vi "SwissSPAD Live_Gate Configuration Storage.vi"(7 "Preset Configuration Refnum":refnum<vi>, 8 "Error In":errorcluster, 9 "Action":T1, 10 "Gate Configuration Definition in":T2, 11 "Gate Configuration Name in":string) -> (0 "Error Out":errorcluster, 1 "Configuration ID":i32, 2 "Gate Configuration Definition out":T2, 3 "Gate Configuration Name out":string, 4 "Gate Configuration Found?":bool, 5 "Gate Definition Found?":bool)   [LabVIEW 2021]
uses:
  SwissSPAD Live_SS2 Gate Configuration.ctl
  SwissSPAD Live_SS2 Gate Definition.ctl
  SwissSPAD Live_Gate Configuration Action.ctl
  SwissSPAD Live_Globals.vi
  <vilib>/UserTags/UserTags.lvlib
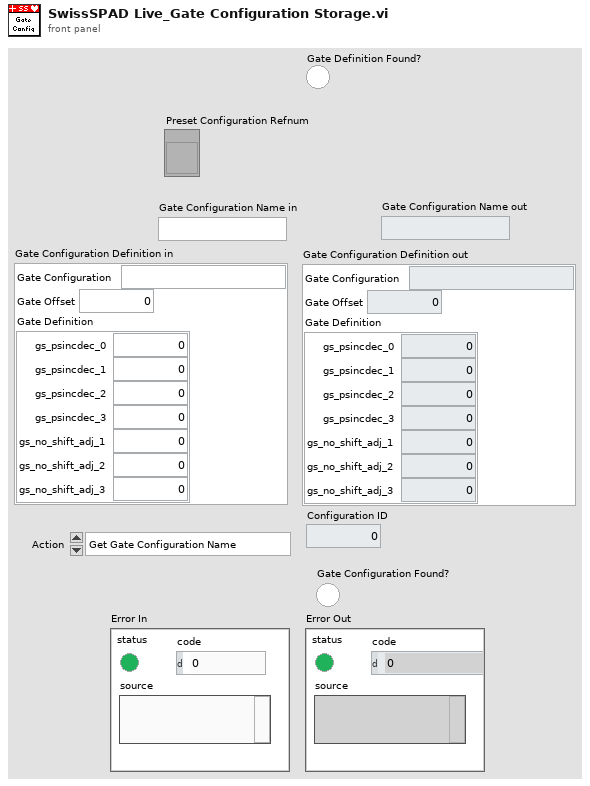
[diagram p1: front panel]
types:
  T1 = typedef "SwissSPAD Live_Gate Configuration Action.ctl" = enum16{"Get Gate Configuration Name", "Get Configuration by Name", "Add Gate Configuration", "Delete Gate Configuration", "Rename Gate Configuration"}
  T2 = typedef "SwissSPAD Live_SS2 Gate Configuration.ctl" = cluster{"Gate Configuration":string, "Gate Offset":u32, "Gate Definition":T3}
  T3 = typedef "SwissSPAD Live_SS2 Gate Definition.ctl" = cluster{"gs_psincdec_0":u32, "gs_psincdec_1":u32, "gs_psincdec_2":u32, "gs_psincdec_3":u32, "gs_no_shift_adj_1":u32, "gs_no_shift_adj_2":u32, "gs_no_shift_adj_3":u32}
  T4 = enum16{"Left Button", "Center Button", "Right Button", "Window Close"}
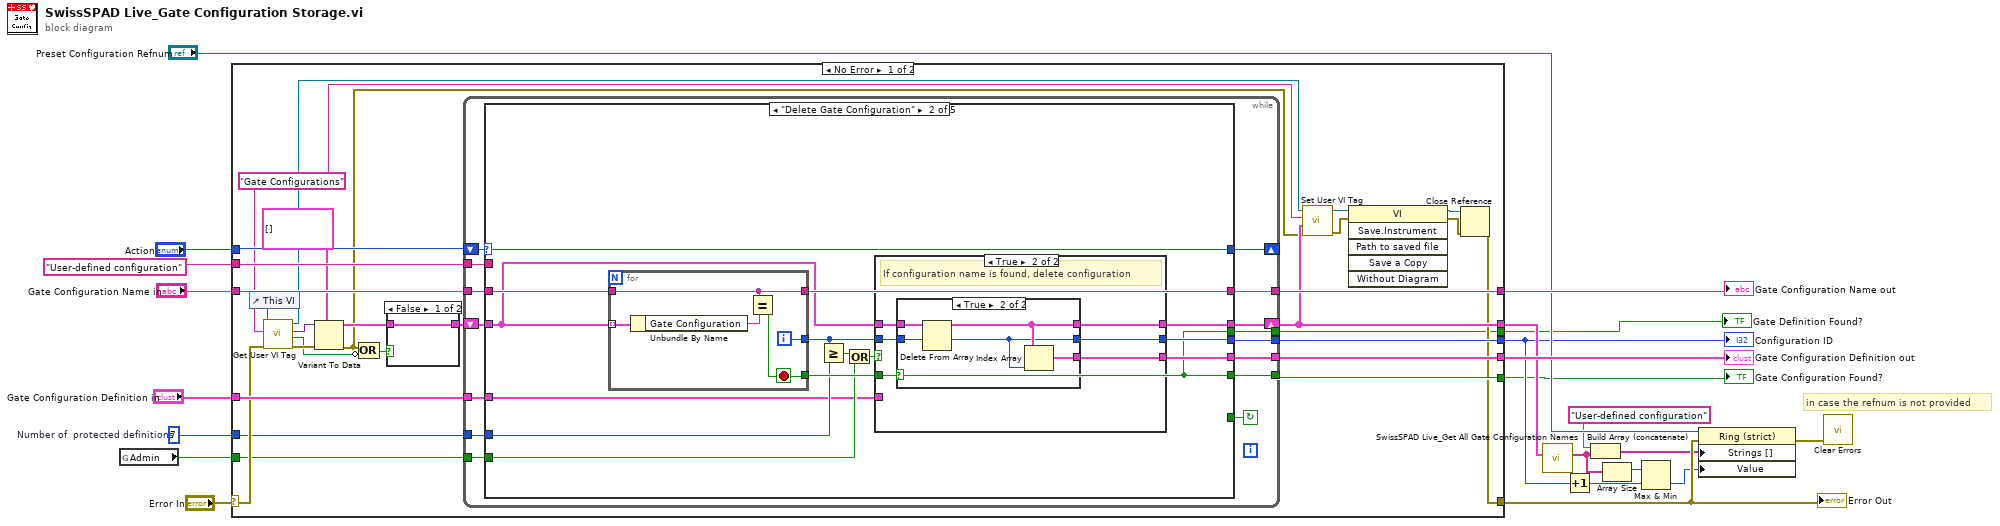
[diagram p0: block diagram]
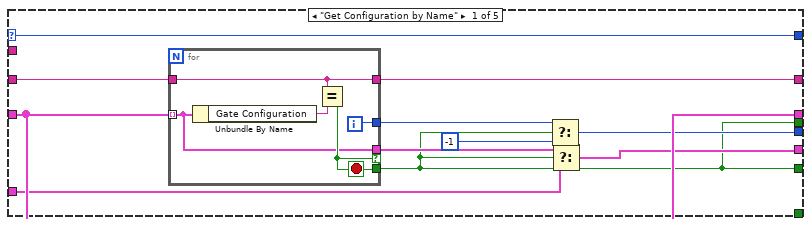
[diagram p3: hidden frame]
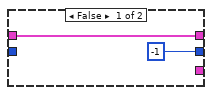
[diagram p5: hidden frame]
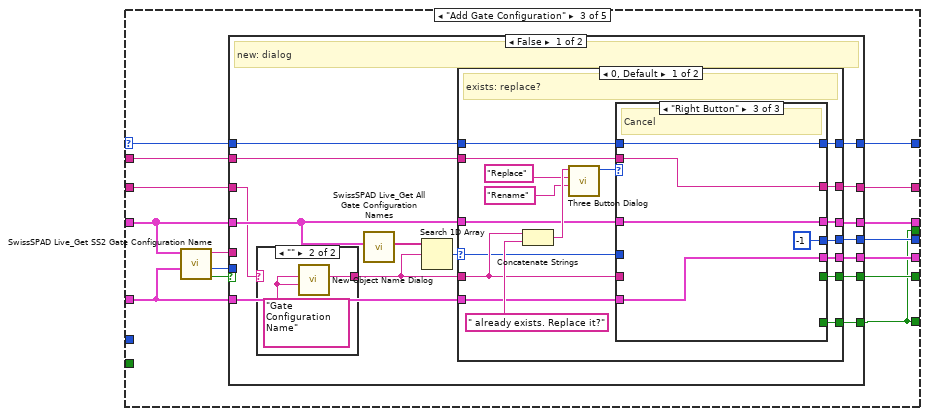
[diagram p6: hidden frame]
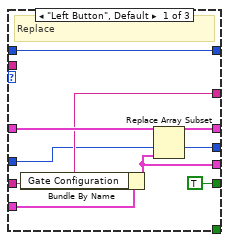
[diagram p8: hidden frame]
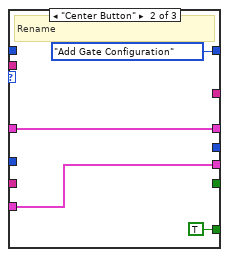
[diagram p9: hidden frame]
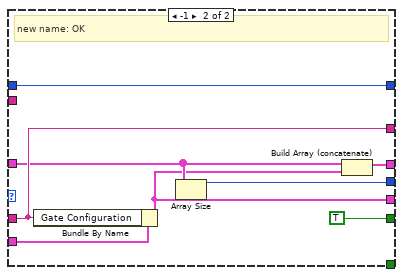
[diagram p10: hidden frame]
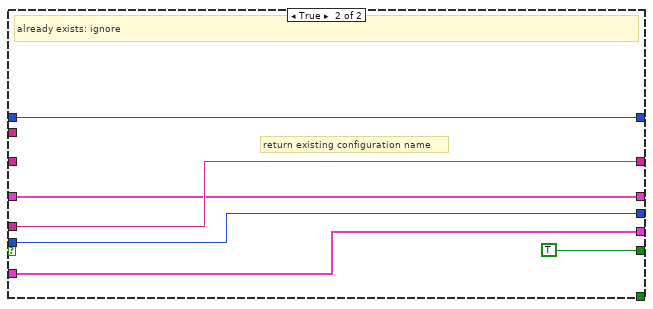
[diagram p11: hidden frame]
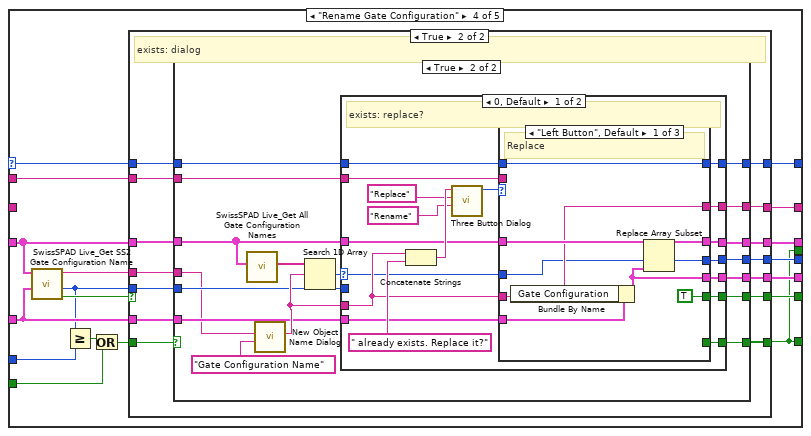
[diagram p12: hidden frame]
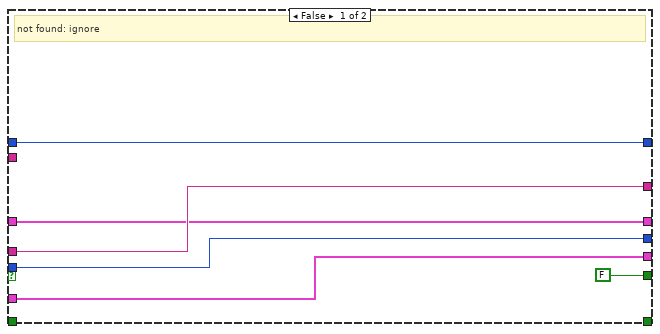
[diagram p13: hidden frame]
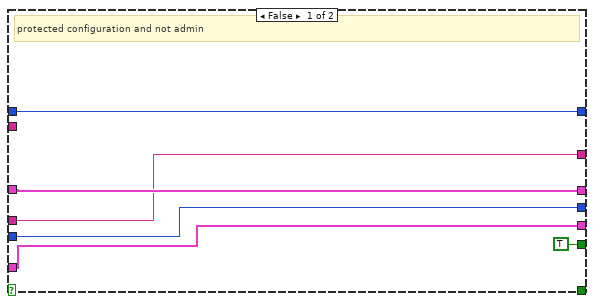
[diagram p14: hidden frame]
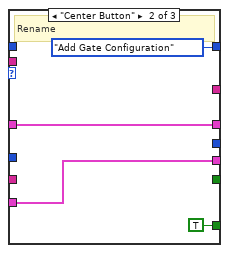
[diagram p15: hidden frame]
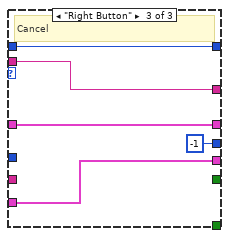
[diagram p16: hidden frame]
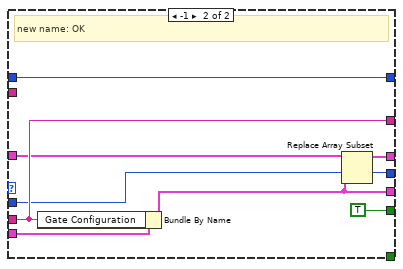
[diagram p17: hidden frame]
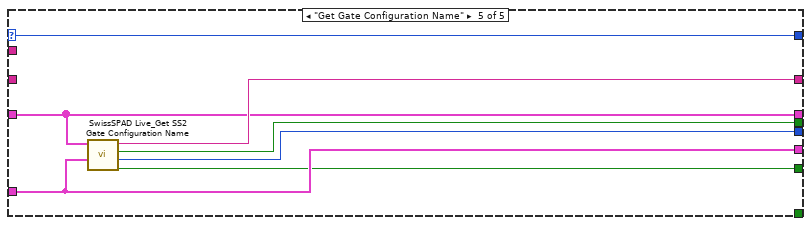
[diagram p18: hidden frame]
diagram:
  w6 = 7  # Number of  protected definitions
  # "in case the refnum is not provided"
  n1 = global read "SwissSPAD Live_Globals.vi" "Admin"() -> (w5:bool)
  n2 = case shown="No Error" "Error In" {
    selector: "Error In" -> [w28 w311]
    tunnel: "Action" -> [w51 _]
    tunnel: "Gate Configuration Name in" -> [w50 _]
    tunnel: [w49 _] -> w20
    tunnel: [w48 _] -> w19
    tunnel: "Gate Configuration Definition in" -> [w47 _]
    tunnel: [w46 _] -> w13
    tunnel: [w45 _] -> w14
    tunnel: "User-defined configuration" ("Object Name out") -> [w44 _]
    tunnel: [w37 _] -> w15
    tunnel: [w26 w311] -> w8
    tunnel: [w25 _] -> w9
    tunnel: w6 -> [w24 _]
    tunnel: w5 -> [w23 _]
    frame No Error {
      w35 = "Gate Configurations" ("Tag Name")
      n3 = control-ref of="This VI"() -> (w43:refnum<vi>)
      n4 = call <vilib>:"Get User VI Tag.vi"("error in (no error)"=w28, "Tag Name"=w35, "VI Refnum"=w43) -> ("error out"=w42:errorcluster, "Was Tag Found?"=w33:bool, "Value"=w41:variant, "dup VI Refnum"=w36:refnum<vi>)  [unwired: 5 in]
      n5 = Variant To Data(error in=w42, type=T2[] [] ("Array"), Variant=w41) -> (data=w39:T2[], error out=w27:errorcluster)
      n6 = Compound Arithmetic op=OR(w27, invert w33) -> (w34:bool)
      n7 = case shown="False" w34 {
        tunnel: w39 -> [w52 _]
        tunnel: [w52 _] -> w38
        frame False {
        }
        frame True {
        }
      }
      n8 = while {
        tunnel: w50 -> [w66]
        shift-right: [w61] -> w37
        shift-left: w38 -> [w65]
        tunnel: [w64] -> w46
        tunnel: [w63] -> w49
        tunnel: [w62] -> w48
        tunnel: w47 -> [w60]
        tunnel: [w59] -> w45
        shift-right: [w58] -> _
        shift-left: w51 -> [w67]
        tunnel: w44 -> [w56]
        tunnel: [w55] -> w25
        tunnel: w24 -> [w54]
        tunnel: w23 -> [w53]
        stop <- w57 continue-if-true
        n9 = case shown="\"Delete Gate Configuration\"" w67 {
          selector: w67 -> [w72 w93 w122 w208 w305]
          tunnel: w66 -> [w78 w97 w119 _ _]
          tunnel: w65 -> [w76 w95 w129 w214 w309]
          tunnel: [w68 w90 w123 w209 w307] -> w64
          tunnel: [w69 w91 w126 w211 w308] -> w63
          tunnel: [w77 w96 w130 w215 w310] -> w62
          tunnel: [w76 w94 w128 w213 w309] -> w61
          tunnel: w60 -> [w70 w84 w127 w212 w308]
          tunnel: [w74 w92 w124 w210 w306] -> w59
          tunnel: [w72 w93 w121 w207 w305] -> w58
          tunnel: [_ _ w118 w205 _] -> w57
          tunnel: w56 -> [_ _ w120 w206 _]
          tunnel: [w68 w90 w118 w205 w304] -> w55
          tunnel: w54 -> [_ w88 _ w202 _]
          tunnel: w53 -> [_ w85 _ w201 _]
          frame "Get Configuration by Name" {
            n10 = for {
              tunnel: w76 -> [w80] mode=indexing
              tunnel: [w82] -> w68
              tunnel: w78 -> [w81]
              tunnel: [w80] -> w71 if=w82
              tunnel: [w81] -> w77
              tunnel: [w79] -> w75
              i -> [w79]
              stop <- w82 stop-if-true
              n11 = Unbundle By Name(w80) -> ("Gate Configuration"=w83:string)
              n12 = Equal?(x=w81, y=w83) -> (x = y?=w82:bool)
            }
            n13 = Select(t=w75, s=w68, f=-1) -> (s? t:f=w74:i32)
            n14 = Select(t=w71, s=w68, f=w70) -> (s? t:f=w69:T2)
          }
          frame "Delete Gate Configuration" {
            n15 = for {
              tunnel: w95 -> [w114] mode=indexing
              tunnel: [w116] -> w90
              tunnel: w97 -> [w115]
              tunnel: [w115] -> w96
              tunnel: [w113] -> w89
              i -> [w113]
              stop <- w116 stop-if-true
              n16 = Unbundle By Name(w114) -> ("Gate Configuration"=w117:string)
              n17 = Equal?(x=w115, y=w117) -> (x = y?=w116:bool)
            }
            n18 = Greater Or Equal?(x=w89, y=w88) -> (x >= y?=w87:bool)
            n19 = Or(x=w87, y=w85) -> (x .or. y?=w86:bool)
            n20 = case shown="True" w86 {
              tunnel: w95 -> [w100 w106]
              tunnel: [w100 w105] -> w94
              tunnel: [w99 w104] -> w92
              tunnel: [w98 w103] -> w91
              tunnel: w90 -> [_ w102]
              tunnel: w89 -> [w99 w101]
              tunnel: w84 -> [w98 _]
              frame False {
                # "protected configuration and not admin"
              }
              frame True {
                # "If configuration name is found, delete configuration"
                n21 = case shown="True" w102 {
                  tunnel: w101 -> [_ w110]
                  tunnel: w106 -> [w108 w112]
                  tunnel: [w108 w111] -> w105
                  tunnel: [-1 w110] -> w104
                  tunnel: [_ w109] -> w103
                  frame False {
                  }
                  frame True {
                    n22 = Delete From Array(array=w112, index=w110) -> (array with subset deleted=w111:T2[])  [unwired: 1 in, 1 out]
                    n23 = Index Array(array=w111, index=w110) -> (element=w109:T2)
                  }
                }
              }
            }
          }
          frame "Add Gate Configuration" {
            n24 = call "SwissSPAD Live_Get SS2 Gate Configuration Name.vi"("Gate Configuration Definition in"=w127, "Gate Configurations Definitions"=w129) -> ("Gate Configuration Found?"=w132:bool, "Configuration ID"=w125:i32, "Gate Configuration Name"=w131:string)  [unwired: 6 in, 1 out]
            n25 = case shown="False" w132 {
              tunnel: w131 -> [_ w199]
              tunnel: [w142 w199] -> w130
              tunnel: w129 -> [w145 w198]
              tunnel: [w141 w198] -> w128
              tunnel: w127 -> [w143 w197]
              tunnel: [w139 w197] -> w126
              tunnel: w125 -> [_ w196]
              tunnel: [w140 w196] -> w124
              tunnel: [w138 TRUE ("Found?")] -> w123
              tunnel: w122 -> [w137 w195]
              tunnel: [w136 w195] -> w121
              tunnel: [w135 _] -> w118
              tunnel: w120 -> [w134 _]
              tunnel: w119 -> [w133 _]
              frame False {
                # "new: dialog"
                n26 = case shown="\"\"" w133 {
                  selector: w133 -> [w148 _]
                  tunnel: [w148 w149] -> w144
                  frame "Name", Default {
                  }
                  frame "" {
                    w150 = "Gate Configuration Name" ("Object Name in")
                    n27 = call "New Object Name Dialog.vi"("String Name (\"object\")"=w150, "Object Name in"=w150) -> ("Object Name out"=w149:string)  [unwired: 7 in, 2 out]
                  }
                }
                n28 = call "SwissSPAD Live_Get All Gate Configuration Names.vi"("Gate Configurations"=w145) -> ("Gate Configuration Names"=w147:string[])  [unwired: 10 in]
                n29 = Search 1D Array(1D array=w147, element=w144) -> (index of element=w146:i32)  [unwired: 1 in]
                n30 = case shown="0, Default" w146 {
                  selector: w146 -> [w156 _]
                  tunnel: w145 -> [w163 w190]
                  tunnel: w144 -> [w159 w192]
                  tunnel: w143 -> [w152 w193]
                  tunnel: [w158 w192] -> w142
                  tunnel: [w162 w191] -> w141
                  tunnel: [w155 w189] -> w140
                  tunnel: [w151 w188] -> w139
                  tunnel: [w154 TRUE ("Found?")] -> w138
                  tunnel: w137 -> [w161 w187]
                  tunnel: [w160 w187] -> w136
                  tunnel: [w157 _] -> w135
                  tunnel: w134 -> [w153 _]
                  frame 0, Default {
                    # "exists: replace?"
                    n31 = Concatenate Strings(w159, " already exists. Replace it?" ("string")) -> (w167:string)
                    n32 = call <vilib>:"Three Button Dialog.vi"("Center Button Text (\"No\")"="Rename" ("F button name (\"Cancel\")"), "Left Button Text (\"Yes\")"="Replace" ("T button name (\"OK\")"), "message"=w167) -> ("Which Button?"=w164:T4)  [unwired: 8 in]
                    n33 = case shown="\"Right Button\"" w164 {
                      tunnel: w163 -> [w175 w179 w185]
                      tunnel: [w172 w179 w185] -> w162
                      tunnel: w161 -> [w173 _ w184]
                      tunnel: [w173 SwissSPAD_Live_Gate_Configuration_Action."Add Gate Configuration" ("Action") w184] -> w160
                      tunnel: w152 -> [w176 w177 w181]
                      tunnel: w159 -> [w174 _ _]
                      tunnel: [w174 _ w183] -> w158
                      tunnel: [_ TRUE _] -> w157
                      tunnel: w156 -> [w171 _ _]
                      tunnel: [w171 _ -1 ("index of element")] -> w155
                      tunnel: [TRUE _ _] -> w154
                      tunnel: w153 -> [_ _ w183]
                      tunnel: [w169 w177 w181] -> w151
                      frame "Left Button", Default {
                        # "Replace"
                        n34 = Bundle By Name(cluster=w176, "Gate Configuration"=w174) -> (w169:T2)
                        n35 = Replace Array Subset(array=w175, new element=w169, index=w171) -> (w172:T2[])
                      }
                      frame "Center Button" {
                        # "Rename"
                      }
                      frame "Right Button" {
                        # "Cancel"
                      }
                    }
                  }
                  frame -1 {
                    # "new name: OK"
                    n36 = Bundle By Name(cluster=w193, "Gate Configuration"=w192) -> (w188:T2)
                    n37 = Array Size(array=w190) -> (size(s)=w189:i32)
                    n38 = Build Array (concatenate)(w190, w188) -> (w191:T2[])
                  }
                }
              }
              frame True {
                # "return existing configuration name"
                # "already exists: ignore"
              }
            }
          }
          frame "Rename Gate Configuration" {
            n39 = call "SwissSPAD Live_Get SS2 Gate Configuration Name.vi"("Gate Configuration Definition in"=w212, "Gate Configurations Definitions"=w214) -> ("Gate Configuration Found?"=w217:bool, "Configuration ID"=w203:i32, "Gate Configuration Name"=w216:string)  [unwired: 6 in, 1 out]
            n40 = Greater Or Equal?(x=w203, y=w202) -> (x >= y?=w204:bool)
            n41 = Or(x=w204, y=w201) -> (x .or. y?=w200:bool)
            n42 = case shown="True" w217 {
              tunnel: w216 -> [w223 w224]
              tunnel: [w223 w235] -> w215
              tunnel: w214 -> [w222 w237]
              tunnel: [w222 w234] -> w213
              tunnel: w212 -> [w221 w236]
              tunnel: [w221 w232] -> w211
              tunnel: w203 -> [w220 w226]
              tunnel: [w220 w233] -> w210
              tunnel: [FALSE ("Found?") w231] -> w209
              tunnel: w208 -> [w219 w230]
              tunnel: [w219 w229] -> w207
              tunnel: [_ w228] -> w205
              tunnel: w206 -> [_ w227]
              tunnel: w200 -> [_ w225]
              frame False {
                # "not found: ignore"
              }
              frame True {
                # "exists: dialog"
                n43 = case shown="True" w225 {
                  tunnel: w237 -> [w240 w257]
                  tunnel: w236 -> [w241 w255]
                  tunnel: [w239 w254] -> w235
                  tunnel: [w240 w253] -> w234
                  tunnel: [w238 w252] -> w233
                  tunnel: [w241 w251] -> w232
                  tunnel: [TRUE ("Found?") w250] -> w231
                  tunnel: w230 -> [w243 w249]
                  tunnel: [w243 w248] -> w229
                  tunnel: [_ w247] -> w228
                  tunnel: w227 -> [_ w246]
                  tunnel: w226 -> [w238 w245]
                  tunnel: w224 -> [w239 w244]
                  frame False {
                    # "protected configuration and not admin"
                  }
                  frame True {
                    n44 = call "SwissSPAD Live_Get All Gate Configuration Names.vi"("Gate Configurations"=w257) -> ("Gate Configuration Names"=w259:string[])  [unwired: 10 in]
                    n45 = call "New Object Name Dialog.vi"("String Name (\"object\")"="Gate Configuration Name" ("Object Name in"), "Object Name in"=w244) -> ("Object Name out"=w256:string)  [unwired: 7 in, 2 out]
                    n46 = Search 1D Array(1D array=w259, element=w256) -> (index of element=w258:i32)  [unwired: 1 in]
                    n47 = case shown="0, Default" w258 {
                      selector: w258 -> [w265 _]
                      tunnel: w257 -> [w273 w300]
                      tunnel: w256 -> [w268 w302]
                      tunnel: w255 -> [w269 w303]
                      tunnel: [w267 w302] -> w254
                      tunnel: [w272 w301] -> w253
                      tunnel: [w264 w296] -> w252
                      tunnel: [w261 w297] -> w251
                      tunnel: [w263 TRUE ("Found?")] -> w250
                      tunnel: w249 -> [w271 w299]
                      tunnel: [w270 w299] -> w248
                      tunnel: [w266 _] -> w247
                      tunnel: w246 -> [w262 _]
                      tunnel: w245 -> [_ w296]
                      frame 0, Default {
                        # "exists: replace?"
                        n48 = Concatenate Strings(w268, " already exists. Replace it?" ("string")) -> (w277:string)
                        n49 = call <vilib>:"Three Button Dialog.vi"("Center Button Text (\"No\")"="Rename" ("F button name (\"Cancel\")"), "Left Button Text (\"Yes\")"="Replace" ("T button name (\"OK\")"), "message"=w277) -> ("Which Button?"=w274:T4)  [unwired: 8 in]
                        n50 = case shown="\"Left Button\", Default" w274 {
                          tunnel: w273 -> [w285 w289 w295]
                          tunnel: [w282 w289 w295] -> w272
                          tunnel: w271 -> [w283 _ w294]
                          tunnel: [w283 SwissSPAD_Live_Gate_Configuration_Action."Add Gate Configuration" ("Action") w294] -> w270
                          tunnel: w269 -> [w286 w287 w291]
                          tunnel: w268 -> [w284 _ _]
                          tunnel: [w284 _ w293] -> w267
                          tunnel: [_ TRUE _] -> w266
                          tunnel: w265 -> [w281 _ _]
                          tunnel: [w281 _ -1 ("index of element")] -> w264
                          tunnel: [TRUE _ _] -> w263
                          tunnel: w262 -> [_ _ w293]
                          tunnel: [w279 w287 w291] -> w261
                          frame "Left Button", Default {
                            # "Replace"
                            n51 = Bundle By Name(cluster=w286, "Gate Configuration"=w284) -> (w279:T2)
                            n52 = Replace Array Subset(array=w285, new element=w279, index=w281) -> (w282:T2[])
                          }
                          frame "Center Button" {
                            # "Rename"
                          }
                          frame "Right Button" {
                            # "Cancel"
                          }
                        }
                      }
                      frame -1 {
                        # "new name: OK"
                        n53 = Bundle By Name(cluster=w303, "Gate Configuration"=w302) -> (w297:T2)
                        n54 = Replace Array Subset(array=w300, new element=w297, index=w296) -> (w301:T2[])
                      }
                    }
                  }
                }
              }
            }
          }
          frame "Get Gate Configuration Name" {
            n55 = call "SwissSPAD Live_Get SS2 Gate Configuration Name.vi"("Gate Configuration Definition in"=w308, "Gate Configurations Definitions"=w309) -> ("Gate Configuration Found?"=w307:bool, "Configuration ID"=w306:i32, "Gate Definition Found?"=w304:bool, "Gate Configuration Name"=w310:string)  [unwired: 6 in]
          }
        }
      }
      n56 = call <vilib>:"Set User VI Tag.vi"("error in (no error)"=w27, "Value"=w37, "Tag Name"=w35, "VI Refnum"=w36) -> ("error out"=w30:errorcluster, "dup VI Refnum"=w32:refnum<vi>)  [unwired: 5 in, 1 out]
      n57 = invoke class="VI" method="Save.Instrument"(reference=w32, error in=w30) -> (reference out=w31:refnum<vi>, error out=w29:errorcluster)  [unwired: 4 in, 4 out]
      n58 = Close Reference(reference=w31, error in (no error)=w29) -> (error out=w26:errorcluster)
    }
    frame Error {
    }
  }
  "Error Out" <- w8
  "Gate Configuration Definition out" <- w20
  "Gate Configuration Name out" <- w19
  "Gate Configuration Found?" <- w13
  "Configuration ID" <- w14
  "Gate Definition Found?" <- w9
  n59 = call "SwissSPAD Live_Get All Gate Configuration Names.vi"("Gate Configurations"=w15) -> ("Gate Configuration Names"=w1:string[])  [unwired: 10 in]
  n60 = Increment(x=w14) -> (x+1=w11:i32)
  n61 = Build Array (concatenate)("User-defined configuration" ("element"), w1) -> (w3:string[])
  n62 = Array Size(array=w1) -> (size(s)=w2:i32)
  n63 = Max & Min(x=w2, y=w11) -> (min(x,y)=w4:i32)  [unwired: 1 out]
  n64 = property class="Ring (strict)"(reference="Preset Configuration Refnum", error in=w8, "Strings []"=w3, "Value"=w4) -> (error out=w7:errorcluster)  [unwired: 1 out]
  n65 = call <vilib>:"Clear Errors.vi"("error in (no error)"=w7) -> ()  [unwired: 5 in, 2 out]
